vi "Move XYZ.vi"(0 "PID Gains In":T1={"X PID"={"proportional gain (Kc)"=0.03, "integral time (Ti, min)"=0.0, "derivative time (Td, min)"=0.0}, "Y PID"={"proportional gain (Kc)"=0.03, "integral time (Ti, min)"=0.0, "derivative time (Td, min)"=0.0}, "Z PID"={"proportional gain (Kc)"=0.035, "integral time (Ti, min)"=0.0, "derivative time (Td, min)"=0.0}} {"Z PID"."derivative time (Td, min)" format="%.3f"; "Z PID"."integral time (Ti, min)" format="%.3f"; "Z PID"."proportional gain (Kc)" format="%.3f"; "Y PID"."derivative time (Td, min)" format="%.3f"; "Y PID"."integral time (Ti, min)" format="%.3f"; "Y PID"."proportional gain (Kc)" format="%.3f"; "X PID"."derivative time (Td, min)" format="%.3f"; "X PID"."integral time (Ti, min)" format="%.3f"; "X PID"."proportional gain (Kc)" format="%.3f"}, 5 "Y Target":dbl, 6 "X Target":dbl, 10 "Max Time":dbl=90.0, 11 "Gyro Target":dbl=-180.0, 12 "Movement":dbl=3.0, 14 "X Output Range":cluster{"output high":dbl, "output low":dbl}={"output high"=0.8, "output low"=-0.8}, 15 "X Stop Threshold":dbl=5.0, 16 "Y Output Range":cluster{"output high":dbl, "output low":dbl}={"output high"=0.8, "output low"=-0.8}, 17 "Y Stop Threshold":dbl=5.0, 18 "Z Output Range":cluster{"output high":dbl, "output low":dbl}={"output high"=0.8, "output low"=-0.8}, 19 "Z  Stop Threshold":dbl=8.0) -> ()   [LabVIEW 2018]
uses:
  Robot Global Data.vi
  SubSystems/Drive Train/Drive Train Global.vi
  <vilib>/addons/control/pid/pid.llb/PID (DBL).vi
  <vilib>/addons/control/pid/NI_PID_pid.lvlib
panel:
  in  "Minimum Time":u32=500
  in  "Settle Time":u32=2000
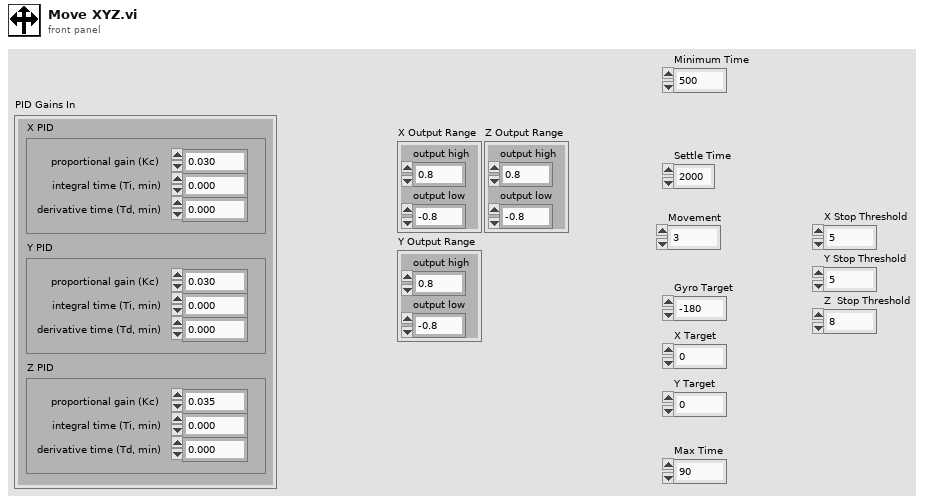
[diagram p1: front panel]
types:
  T1 = cluster{"X PID":cluster{"proportional gain (Kc)":dbl, "integral time (Ti, min)":dbl, "derivative time (Td, min)":dbl}, "Y PID":cluster{"proportional gain (Kc)":dbl, "integral time (Ti, min)":dbl, "derivative time (Td, min)":dbl}, "Z PID":cluster{"proportional gain (Kc)":dbl, "integral time (Ti, min)":dbl, "derivative time (Td, min)":dbl}}
  T2 = cluster{"proportional gain (Kc)":dbl, "integral time (Ti, min)":dbl, "derivative time (Td, min)":dbl}
  T3 = cluster{"Rollover":dbl, "Yaw":dbl, "Cont Yaw":dbl}
  T4 = cluster{"offsetAngle H":dbl, "offsetAngle V":dbl, "area":dbl, "skew":dbl, "validTarget":dbl, "latency":dbl}
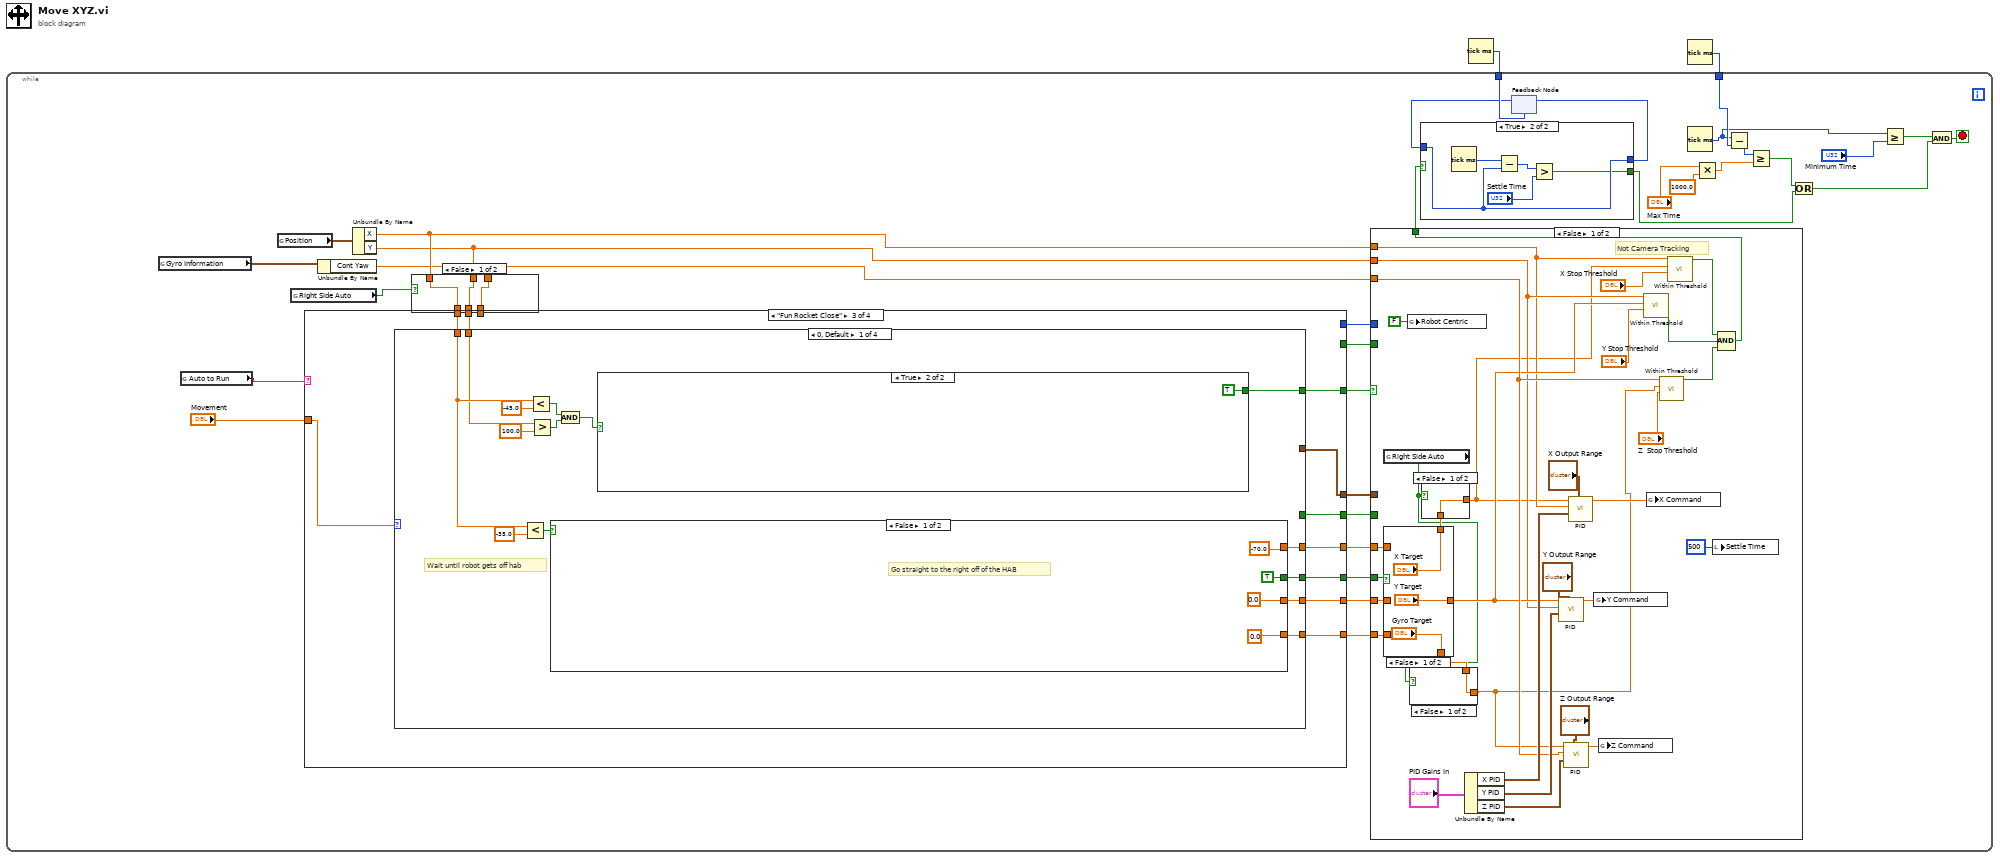
[diagram p0: block diagram]
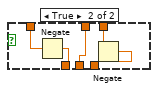
[diagram p2: hidden frame]
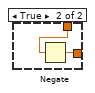
[diagram p3: hidden frame]
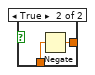
[diagram p4: hidden frame]
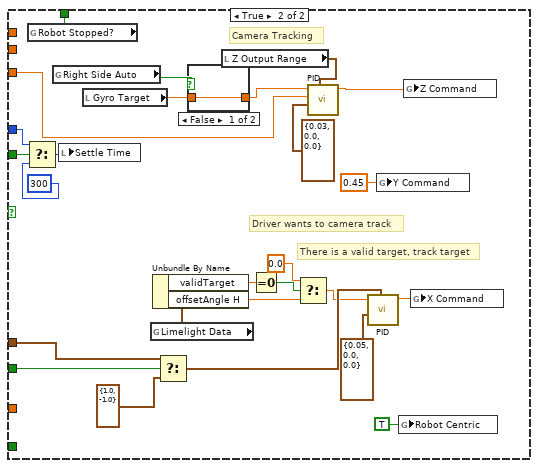
[diagram p6: hidden frame]
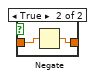
[diagram p7: hidden frame]
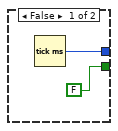
[diagram p8: hidden frame]
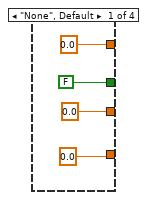
[diagram p9: hidden frame]
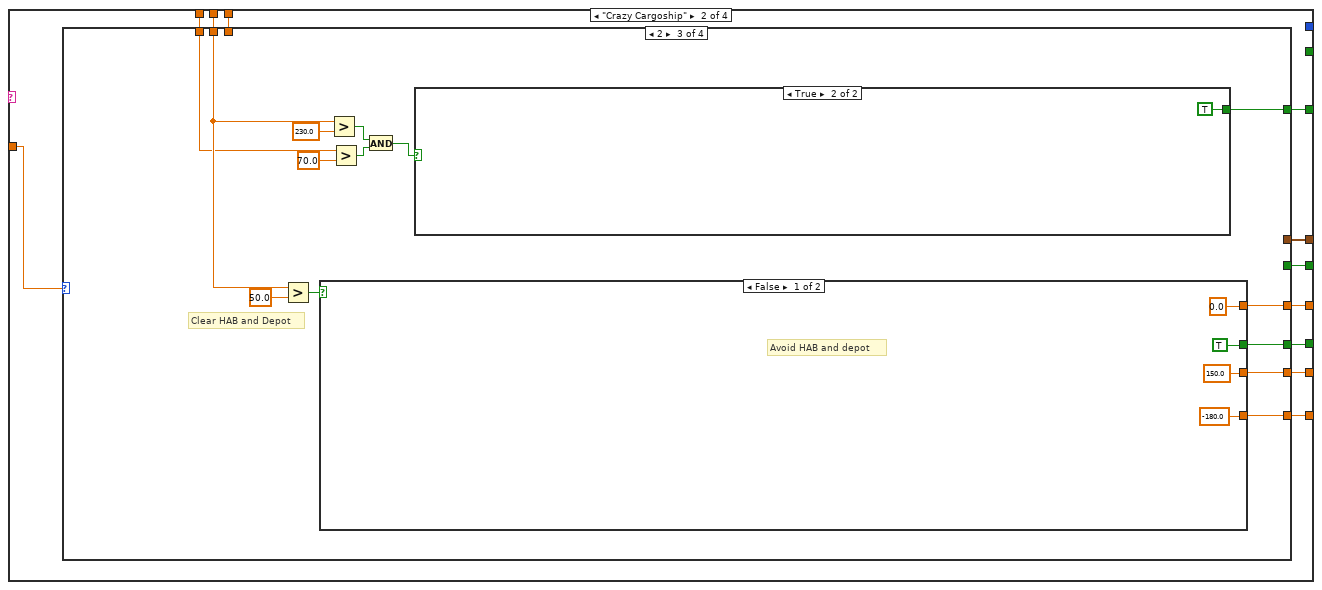
[diagram p10: hidden frame]
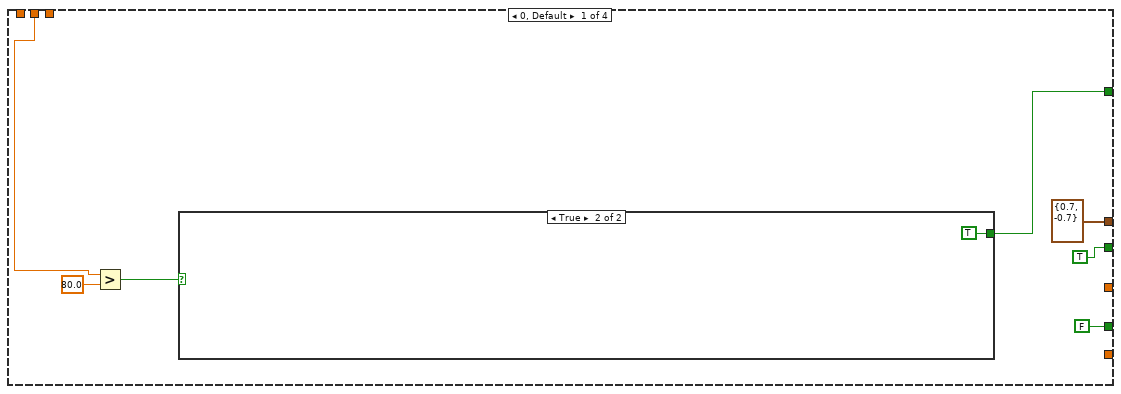
[diagram p11: hidden frame]
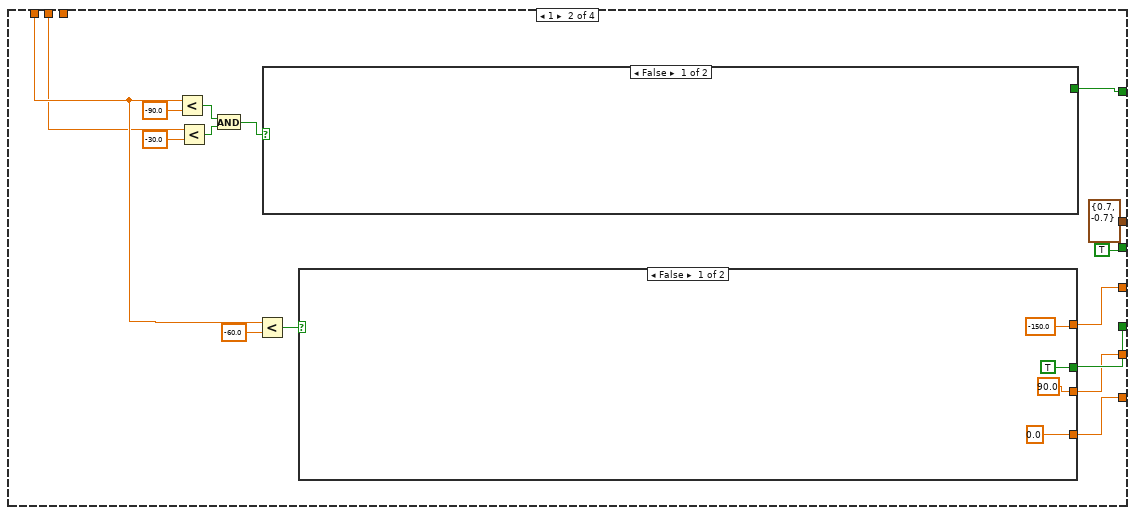
[diagram p13: hidden frame]
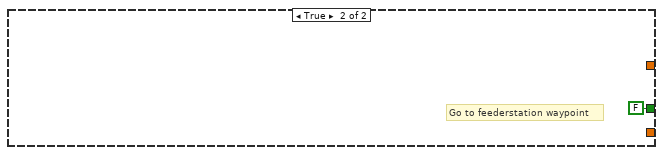
[diagram p14: hidden frame]
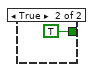
[diagram p15: hidden frame]
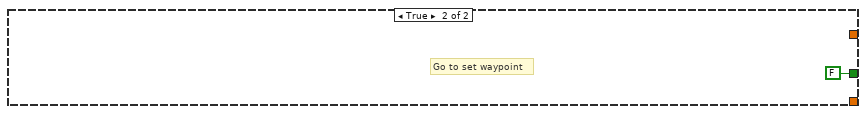
[diagram p17: hidden frame]
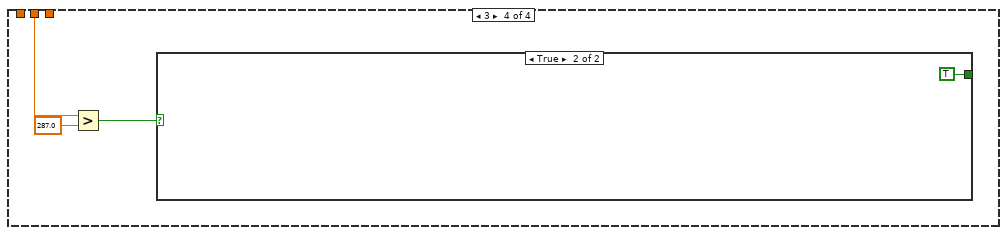
[diagram p18: hidden frame]
diagram:
  n1 = Tick Count (ms)() -> (millisecond timer value=w2:u32)
  n2 = Tick Count (ms)() -> (millisecond timer value=w1:u32)
  n3 = while {
    tunnel: w2 -> [w32]
    tunnel: w1 -> [w20]
    stop <- w19 stop-if-true
    n4 = global read "Drive Train Global.vi" "Gyro Information"() -> (w26:T3)
    n5 = global read "Robot Global Data.vi" "Auto to Run"() -> (w29:string)
    n6 = global read "Drive Train Global.vi" "Position"() -> (w28:cluster{"X":dbl, "Y":dbl})
    n7 = global read "Robot Global Data.vi" "Right Side Auto"() -> (w3:bool)
    n8 = Unbundle By Name(w26) -> ("Cont Yaw"=w5:dbl)
    n9 = Unbundle By Name(w28) -> ("X"=w8:dbl, "Y"=w6:dbl)
    n10 = case shown="False" w3 {
      tunnel: [w41 w46] -> w9
      tunnel: w8 -> [w41 w45]
      tunnel: [w40 w44] -> w7
      tunnel: w6 -> [w40 w44]
      tunnel: w5 -> [w39 w43]
      tunnel: [w39 w42] -> w4
      frame False {
      }
      frame True {
        n11 = Negate(x=w45) -> (-x=w46:dbl)
        n12 = Negate(x=w43) -> (-x=w42:dbl)
      }
    }
    n13 = case shown="\"Fun Rocket Close\"" w29 {
      tunnel: [0.0 w136 w201 w276] -> w38
      tunnel: [0.0 w135 w200 w275] -> w37
      tunnel: [0.0 w134 w199 w274] -> w36
      tunnel: w7 -> [_ w140 w204 w279]
      tunnel: [FALSE w139 w202 w277] -> w35
      tunnel: w9 -> [_ w137 w203 w278]
      tunnel: "Movement" -> [_ w141 w205 w280]
      tunnel: w4 -> [_ w138 _ w272]
      tunnel: [_ w133 w198 w273] -> w14
      tunnel: [_ w131 w196 _] -> w13
      tunnel: [_ w132 w197 _] -> w12
      tunnel: [_ _ _ w271] -> w11
      tunnel: [_ _ _ w270] -> w10
      frame "None", Default {
      }
      frame "Crazy Cargoship" {
        n14 = case shown="2" w141 {
          tunnel: w140 -> [w144 w154 w173 w192]
          tunnel: [FALSE w165 w185 _] -> w139
          tunnel: w138 -> [_ _ _ _]
          tunnel: w137 -> [_ w155 w172 _]
          tunnel: [_ w164 w182 _] -> w136
          tunnel: [_ w163 w181 _] -> w135
          tunnel: [_ w162 w180 _] -> w134
          tunnel: [w146 w156 w174 _] -> w133
          tunnel: [TRUE ("Robot Centric") TRUE ("Robot Centric") _ _] -> w132
          tunnel: [cluster{"output high":dbl, "output low":dbl} {"output high"=0.7, "output low"=-0.7} ("output range") cluster{"output high":dbl, "output low":dbl} {"output high"=0.7, "output low"=-0.7} ("output range") _ _] -> w131
          frame 0, Default {
            n15 = Greater?(x=w144, y=80.0) -> (0:w145:bool)
            n16 = case shown="True" w145 {
              tunnel: [_ TRUE] -> w146
              frame False {
              }
              frame True {
              }
            }
          }
          frame 1 {
            n17 = Less?(x=w155, y=-90.0) -> (x < y?=w159:bool)
            n18 = Less?(x=w154, y=-30.0) -> (x < y?=w158:bool)
            n19 = And(x=w159, y=w158) -> (x .and. y?=w157:bool)
            n20 = Less?(x=w155, y=-60.0) -> (x < y?=w150:bool)
            n21 = case shown="False" w157 {
              tunnel: [_ TRUE] -> w156
              frame False {
              }
              frame True {
              }
            }
            n22 = case shown="False" w150 {
              tunnel: [TRUE FALSE] -> w165
              tunnel: [-150.0 _] -> w164
              tunnel: [90.0 _] -> w163
              tunnel: [0.0 _] -> w162
              frame False {
              }
              frame True {
                # "Go to feederstation waypoint"
              }
            }
          }
          frame 2 {
            # "Clear HAB and Depot"
            n23 = Greater?(x=w173, y=50.0) -> (0:w184:bool)
            n24 = case shown="False" w184 {
              tunnel: [TRUE FALSE] -> w185
              tunnel: [0.0 _] -> w182
              tunnel: [150.0 _] -> w181
              tunnel: [-180.0 _] -> w180
              frame False {
                # "Avoid HAB and depot"
              }
              frame True {
                # "Go to set waypoint"
              }
            }
            n25 = Greater?(x=w173, y=230.0) -> (0:w177:bool)
            n26 = Greater?(x=w172, y=70.0) -> (0:w176:bool)
            n27 = And(x=w177, y=w176) -> (x .and. y?=w175:bool)
            n28 = case shown="True" w175 {
              tunnel: [_ TRUE] -> w174
              frame False {
              }
              frame True {
              }
            }
          }
          frame 3 {
            n29 = Greater?(x=w192, y=287.0) -> (0:w193:bool)
            n30 = case shown="True" w193 {
              tunnel: [_ TRUE] -> _
              frame False {
              }
              frame True {
              }
            }
          }
        }
      }
      frame "Fun Rocket Close" {
        n31 = case shown="0, Default" w205 {
          tunnel: w204 -> [w212 w226 w239 w260]
          tunnel: w203 -> [w213 w227 _ _]
          tunnel: [w217 _ w237 w255] -> w202
          tunnel: [w216 _ w238 w258] -> w201
          tunnel: [w215 _ w236 w257] -> w200
          tunnel: [w214 _ w235 w256] -> w199
          tunnel: [w206 w228 w245 w263] -> w198
          tunnel: [_ _ w243 _] -> w197
          tunnel: [_ _ w242 _] -> w196
          frame 0, Default {
            # "Wait until robot gets off hab"
            n32 = Less?(x=w213, y=-35.0) -> (x < y?=w219:bool)
            n33 = Less?(x=w213, y=-45.0) -> (x < y?=w209:bool)
            n34 = Greater?(x=w212, y=100.0) -> (0:w208:bool)
            n35 = case shown="False" w219 {
              tunnel: [TRUE FALSE] -> w217
              tunnel: [-70.0 _] -> w216
              tunnel: [0.0 _] -> w215
              tunnel: [0.0 _] -> w214
              frame False {
                # "Go straight to the right off of the HAB"
              }
              frame True {
                # "Robot off of HAB, go to the rocket"
              }
            }
            n36 = And(x=w209, y=w208) -> (x .and. y?=w207:bool)
            n37 = case shown="True" w207 {
              tunnel: [_ TRUE] -> w206
              frame False {
              }
              frame True {
              }
            }
          }
          frame 1 {
            n38 = Less?(x=w226, y=-17.0) -> (x < y?=w231:bool)
            n39 = Less?(x=w227, y=-90.0) -> (x < y?=w230:bool)
            n40 = And(x=w231, y=w230) -> (x .and. y?=w229:bool)
            n41 = case shown="True" w229 {
              tunnel: [_ TRUE] -> w228
              frame False {
              }
              frame True {
              }
            }
          }
          frame 2 {
            # "back up then turn"
            n42 = Greater?(x=w239, y=150.0) -> (0:w244:bool)
            n43 = Greater?(x=w239, y=40.0) -> (0:w240:bool)
            n44 = case shown="True" w244 {
              tunnel: [_ TRUE] -> w245
              tunnel: [_ TRUE] -> w243
              tunnel: [_ cluster{"output high":dbl, "output low":dbl} {"output high"=0.6, "output low"=-0.6} ("output range")] -> w242
              frame False {
              }
              frame True {
              }
            }
            n45 = case shown="False" w240 {
              tunnel: [0.0 _] -> w238
              tunnel: [TRUE FALSE] -> w237
              tunnel: [200.0 _] -> w236
              tunnel: [-180.0 _] -> w235
              frame False {
              }
              frame True {
              }
            }
          }
          frame 3 {
            n46 = Less?(x=w260, y=30.0) -> (x < y?=w262:bool)
            n47 = Less?(x=w260, y=140.0) -> (x < y?=w259:bool)
            n48 = case shown="True" w259 {
              tunnel: [0.0 _] -> w258
              tunnel: [100.0 _] -> w257
              tunnel: [-30.0 _] -> w256
              tunnel: [TRUE _] -> w255
              frame False {
              }
              frame True {
              }
            }
            n49 = case shown="False" w262 {
              tunnel: [_ TRUE] -> w263
              frame False {
              }
              frame True {
              }
            }
          }
        }
      }
      frame "Fun Rocket Far" {
        n50 = case shown="2" w280 {
          tunnel: w279 -> [w286 w316 w351 w367]
          tunnel: w278 -> [w285 w323 _ _]
          tunnel: [w291 w321 w356 w362] -> w277
          tunnel: [w290 w322 w355 w365] -> w276
          tunnel: [w289 w320 w354 w364] -> w275
          tunnel: [w288 w319 w353 w363] -> w274
          tunnel: [w287 w325 _ w370] -> w273
          tunnel: w272 -> [_ _ _ _]
          tunnel: [w283 _ _ _] -> w271
          tunnel: [w284 _ _ _] -> w270
          frame 0, Default {
            # "Move to far rocket"
            # "Wait until robot gets off hab"
            n51 = Greater?(x=w286, y=210.0) -> (0:w281:bool)
            n52 = call "Flip Lock.vi"("Input"=w281) -> ("Output"=w282:bool)  [unwired: 10 in]
            n53 = case shown="True" w282 {
              tunnel: [TRUE w307] -> w291
              tunnel: [-10.0 w306] -> w290
              tunnel: [250.0 w305] -> w289
              tunnel: [0.0 w304] -> w288
              tunnel: [_ w303] -> w287
              tunnel: w285 -> [_ w301]
              tunnel: [_ w298] -> w284
              tunnel: [_ w297] -> w283
              frame False {
              }
              frame True {
                # "Wait for robot to be in good\nplace to camera track"
                n54 = Less?(x=w301, y=-80.0) -> (x < y?=w300:bool)
                n55 = call "Flip Lock.vi"("Input"=w300) -> ("Output"=w299:bool)  [unwired: 10 in]
                n56 = case shown="False" w299 {
                  tunnel: [TRUE FALSE] -> w307
                  tunnel: [-150.0 ("y") _] -> w306
                  tunnel: [230.0 ("y") _] -> w305
                  tunnel: [-130.0 ("y") _] -> w304
                  tunnel: [FALSE w313] -> w303
                  tunnel: [_ u32 500 ("Settle Time")] -> w298
                  tunnel: [_ w313] -> w297
                  frame False {
                  }
                  frame True {
                    w313 = TRUE
                  }
                }
              }
            }
          }
          frame 1 {
            n57 = Less?(x=w316, y=-30.0) -> (x < y?=w328:bool)
            n58 = Less?(x=w323, y=0.0) -> (x < y?=w327:bool)
            n59 = And(x=w328, y=w327) -> (x .and. y?=w326:bool)
            n60 = Greater?(x=w323, y=-60.0) -> (0:w317:bool)
            n61 = case shown="False" w326 {
              tunnel: [FALSE TRUE] -> w325
              frame False {
              }
              frame True {
              }
            }
            n62 = call "Flip Lock.vi"("Input"=w317) -> ("Output"=w318:bool)  [unwired: 10 in]
            n63 = case shown="True" w318 {
              tunnel: [0.0 ("y") w337] -> w322
              tunnel: [TRUE w338] -> w321
              tunnel: [230.0 ("y") w336] -> w320
              tunnel: [-150.0 ("y") w335] -> w319
              tunnel: w316 -> [_ w340]
              frame False {
              }
              frame True {
                n64 = Less?(x=w340, y=40.0) -> (x < y?=w341:bool)
                n65 = call "Flip Lock.vi"("Input"=w341) -> ("Output"=w342:bool)  [unwired: 10 in]
                n66 = case shown="True" w342 {
                  tunnel: [TRUE FALSE] -> w338
                  tunnel: [-70.0 ("y") _] -> w337
                  tunnel: [-40.0 ("y") _] -> w336
                  tunnel: [-180.0 ("y") _] -> w335
                  frame False {
                  }
                  frame True {
                  }
                }
              }
            }
          }
          frame 2 {
            n67 = Less?(x=w351, y=30.0) -> (x < y?=w352:bool)
            n68 = case shown="False" w352 {
              tunnel: [TRUE FALSE] -> w356
              tunnel: [-30.0 _] -> w355
              tunnel: [100.0 _] -> w354
              tunnel: [-180.0 _] -> w353
              frame False {
              }
              frame True {
              }
            }
          }
          frame 3 {
            n69 = Less?(x=w367, y=30.0) -> (x < y?=w369:bool)
            n70 = Less?(x=w367, y=140.0) -> (x < y?=w366:bool)
            n71 = case shown="False" w366 {
              tunnel: [0.0 _] -> w365
              tunnel: [100.0 _] -> w364
              tunnel: [-30.0 _] -> w363
              tunnel: [TRUE _] -> w362
              frame False {
              }
              frame True {
              }
            }
            n72 = case shown="True" w369 {
              tunnel: [_ TRUE] -> w370
              frame False {
              }
              frame True {
              }
            }
          }
        }
      }
    }
    n73 = case shown="False" w14 {
      tunnel: w38 -> [w71 _]
      tunnel: w37 -> [w70 _]
      tunnel: w36 -> [w69 _]
      tunnel: w35 -> [w68 _]
      tunnel: [w54 w104] -> w25
      tunnel: w5 -> [w63 w110]
      tunnel: w6 -> [w59 _]
      tunnel: w8 -> [w56 _]
      tunnel: w13 -> [_ w106]
      tunnel: w12 -> [_ w105]
      tunnel: w11 -> [_ w101]
      tunnel: w10 -> [_ w100]
      frame False {
        # "Not Camera Tracking"
        n74 = global read "Robot Global Data.vi" "Right Side Auto"() -> (w47:bool)
        n75 = case shown="False" w68 {
          tunnel: ["X Target" w90] -> w51
          tunnel: ["Y Target" w89] -> w60
          tunnel: ["Gyro Target" w88] -> w49
          tunnel: w71 -> [_ w90]
          tunnel: w70 -> [_ w89]
          tunnel: w69 -> [_ w88]
          frame False {
          }
          frame True {
          }
        }
        n76 = global write "Drive Train Global.vi" "Robot Centric"(FALSE ("Robot Centric")) -> ()
        n77 = case shown="False" w47 {
          tunnel: w49 -> [w79 w80]
          tunnel: [w79 w81] -> w48
          frame False {
          }
          frame True {
            n78 = Negate(x=w80) -> (-x=w81:dbl)
          }
        }
        n79 = case shown="False" w47 {
          tunnel: w51 -> [w82 w83]
          tunnel: [w82 w84] -> w50
          frame False {
          }
          frame True {
            n80 = Negate(x=w83) -> (-x=w84:dbl)
          }
        }
        n81 = Unbundle By Name("PID Gains In") -> ("X PID"=w76:T2, "Y PID"=w75:T2, "Z PID"=w74:T2)
        n82 = call-poly <vilib>:"PID.vi"("output range"="Y Output Range", "PID gains"=w75, "process variable"=w59, "setpoint"=w60) -> ("output"=w65:dbl)  [unwired: 6 in, 1 out]
        n83 = call-poly <vilib>:"PID.vi"("output range"="Z Output Range", "PID gains"=w74, "process variable"=w63, "setpoint"=w48) -> ("output"=w66:dbl)  [unwired: 6 in, 1 out]
        n84 = call-poly <vilib>:"PID.vi"("output range"="X Output Range", "PID gains"=w76, "process variable"=w56, "setpoint"=w50) -> ("output"=w67:dbl)  [unwired: 6 in, 1 out]
        n85 = global write "Drive Train Global.vi" "Y Command"(w65) -> ()
        n86 = global write "Drive Train Global.vi" "Z Command"(w66) -> ()
        n87 = call "Within Threshold.vi"("Threshold"="Y Stop Threshold", "Center"=w60, "Value"=w59) -> ("Within Threshold?"=w61:bool)  [unwired: 8 in]
        n88 = global write "Drive Train Global.vi" "X Command"(w67) -> ()
        n89 = call "Within Threshold.vi"("Threshold"="Z  Stop Threshold", "Center"=w48, "Value"=w63) -> ("Within Threshold?"=w64:bool)  [unwired: 8 in]
        n90 = call "Within Threshold.vi"("Threshold"="X Stop Threshold", "Center"=w50, "Value"=w56) -> ("Within Threshold?"=w57:bool)  [unwired: 8 in]
        n91 = local write "Settle Time"(u32 500 ("Settle Time")) -> ()
        n92 = Compound Arithmetic op=AND(w57, w61, w64) -> (w54:bool)
      }
      frame True {
        # "There is a valid target, track target"
        # "Driver wants to camera track"
        # "Camera Tracking"
        n93 = Select(t=w100, s=w101, f=u32 300 ("Settle Time")) -> (s? t:f=w103:u32)
        n94 = global read "Drive Train Global.vi" "Robot Stopped?"() -> (w104:bool)
        n95 = global read "Robot Global Data.vi" "Right Side Auto"() -> (w92:bool)
        n96 = local write "Settle Time"(w103) -> ()
        n97 = local read "Gyro Target"() -> (w94:dbl)
        n98 = global read "Robot Global Data.vi" "Limelight Data"() -> (w114:T4)
        n99 = Unbundle By Name(w114) -> ("validTarget"=w99:dbl, "offsetAngle H"=w98:dbl)
        n100 = Select(t=w106, s=w105, f=cluster{"output high":dbl, "output low":dbl} {"output high"=1.0, "output low"=-1.0} ("output range")) -> (s? t:f=w107:cluster{"output high":dbl, "output low":dbl})
        n101 = case shown="False" w92 {
          tunnel: w94 -> [w117 w118]
          tunnel: [w117 w119] -> w93
          frame False {
          }
          frame True {
            n102 = Negate(x=w118) -> (-x=w119:dbl)
          }
        }
        n103 = local read "Z Output Range"() -> (w111:cluster{"output high":dbl, "output low":dbl})
        n104 = Equal To 0?(x=w99) -> (x = 0?=w96:bool)
        n105 = Select(t=0.0, s=w96, f=w98) -> (s? t:f=w97:dbl)
        n106 = call-poly <vilib>:"PID.vi"("output range"=w111, "PID gains"=T2 {"proportional gain (Kc)"=0.03, "integral time (Ti, min)"=0.0, "derivative time (Td, min)"=0.0}, "process variable"=w110, "setpoint"=w93) -> ("output"=w91:dbl)  [unwired: 6 in, 1 out]
        n107 = call-poly <vilib>:"PID.vi"("output range"=w107, "PID gains"=T2 {"proportional gain (Kc)"=0.05, "integral time (Ti, min)"=0.0, "derivative time (Td, min)"=0.0} ("Camera Tracking"), "setpoint"=w97) -> ("output"=w115:dbl)  [unwired: 7 in, 1 out]
        n108 = global write "Drive Train Global.vi" "Y Command"(0.45 ("Y Command")) -> ()
        n109 = global write "Drive Train Global.vi" "Robot Centric"(TRUE ("Robot Centric")) -> ()
        n110 = global write "Drive Train Global.vi" "Z Command"(w91) -> ()
        n111 = global write "Drive Train Global.vi" "X Command"(w115) -> ()
      }
    }
    n112 = feedback #1(w32) -> (w31:u32)
    n113 = case shown="True" w25 {
      tunnel: [w121 w124] -> w33
      tunnel: w31 -> [_ w124]
      tunnel: [FALSE w123] -> w30
      frame False {
        n114 = Tick Count (ms)() -> (millisecond timer value=w121:u32)
      }
      frame True {
        n115 = Tick Count (ms)() -> (millisecond timer value=w126:u32)
        n116 = Subtract(x=w126, y=w124) -> (x-y=w125:u32)
        n117 = Greater?(x=w125, y="Settle Time") -> (0:w123:bool)
      }
    }
    n118 = feedback-in #1(w33) -> ()
    n119 = Tick Count (ms)() -> (millisecond timer value=w18:u32)
    n120 = Multiply(x="Max Time", y=1000.0) -> (x*y=w23:dbl)
    n121 = Subtract(x=w18, y=w20) -> (x-y=w24:u32)
    n122 = Greater Or Equal?(x=w24, y=w23) -> (x >= y?=w34:bool)
    n123 = Or(x=w34, y=w30) -> (x .or. y?=w15:bool)
    n124 = Greater Or Equal?(x=w18, y="Minimum Time") -> (x >= y?=w16:bool)
    n125 = And(x=w16, y=w15) -> (x .and. y?=w19:bool)
  }
